vi "test Configuration File Read and Write.vi"(8 "error in (no error)":errorcluster, 11 "TestCase in":refnum<class "Configuration Tests.lvclass">) -> (0 "error out":errorcluster, 3 "TestCase out":refnum<class "Configuration Tests.lvclass">)   [LabVIEW 2017, in "Configuration Tests.lvclass"]
uses:
  Configuration Tests.lvclass
  Typedefs/DSF Engine Framework Configuration.ctl
  Typedefs/DSF Engine Plugin Configuration.ctl
  Typedefs/DSF Timing Info.ctl
  Typedefs/DSF Engine Plugin Thread Configuration.ctl
  Typedefs/DSF Settings Info.ctl
  Typedefs/DSF Engine Transfer Group Configuration.ctl
  Typedefs/DSF Direction.ctl
  Typedefs/DSF Engine Transfer Configuration.ctl
  Typedefs/DSF Byte Order.ctl
  Typedefs/DSF Engine Channel Configuration.ctl
  Typedefs/DSF Data Type.ctl
  Typedefs/DSF Timeout Behavior.ctl
  <vilib>/addons/_JKI Toolkits/VI Tester/TestCase.llb/TestCase.lvclass
  Classes/Configuration/Configuration Session.lvclass
  DSF Core.lvlib
  C:/Program Files (x86)/National Instruments/LabVIEW 2017/vi.lib/addons/_JKI Toolkits/VI Tester/TestCase.llb/TestCase.lvclass
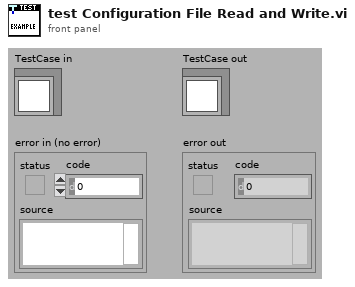
[diagram p1: front panel]
types:
  T1 = typedef "DSF Core.lvlib/DSF Engine Framework Configuration.ctl" = cluster{"Plugins":T2[]}
  T2 = typedef "DSF Core.lvlib/DSF Engine Plugin Configuration.ctl" = cluster{"name":string, "components":string[], "cycle timing":T3, "threads":T4[], "Transfer Groups":T6[], "settings":T5}
  T3 = typedef "DSF Core.lvlib/DSF Timing Info.ctl" = cluster{"priority":u64, "decimation":u64, "offset":u64}
  T4 = typedef "DSF Core.lvlib/DSF Engine Plugin Thread Configuration.ctl" = cluster{"buffer converter settings":T5, "transceiver settings":T5, "processor":i32, "priority offset":i16}
  T5 = typedef "DSF Core.lvlib/DSF Settings Info.ctl" = cluster{"key":string, "value":string}[]
  T6 = typedef "DSF Core.lvlib/DSF Engine Transfer Group Configuration.ctl" = cluster{"name":string, "direction":T7, "cycle timing":T3, "thread index":i32, "settings":T5, "Transfers":T8[], "timeout behavior":T12}
  T7 = typedef "DSF Core.lvlib/DSF Direction.ctl" = enum8{"Tx", "Rx"}
  T8 = typedef "DSF Core.lvlib/DSF Engine Transfer Configuration.ctl" = cluster{"name":string, "byte order":T9, "settings":T5, "channels":T10[]}
  T9 = typedef "DSF Core.lvlib/DSF Byte Order.ctl" = enum8{"big-endian", "little-endian"}
  T10 = typedef "DSF Core.lvlib/DSF Engine Channel Configuration.ctl" = cluster{"string offset":u64, "string data type":T11, "engine data type":T11, "name":string, "settings":T5, "units":string}
  T11 = typedef "DSF Core.lvlib/DSF Data Type.ctl" = enum8{"Bool", "SGL", "DBL", "I8", "I16", "I32", "I64", "U8", "U16", "U32", "U64"}
  T12 = typedef "DSF Core.lvlib/DSF Timeout Behavior.ctl" = enum8{"Increment Late Count", "Throw Error"}
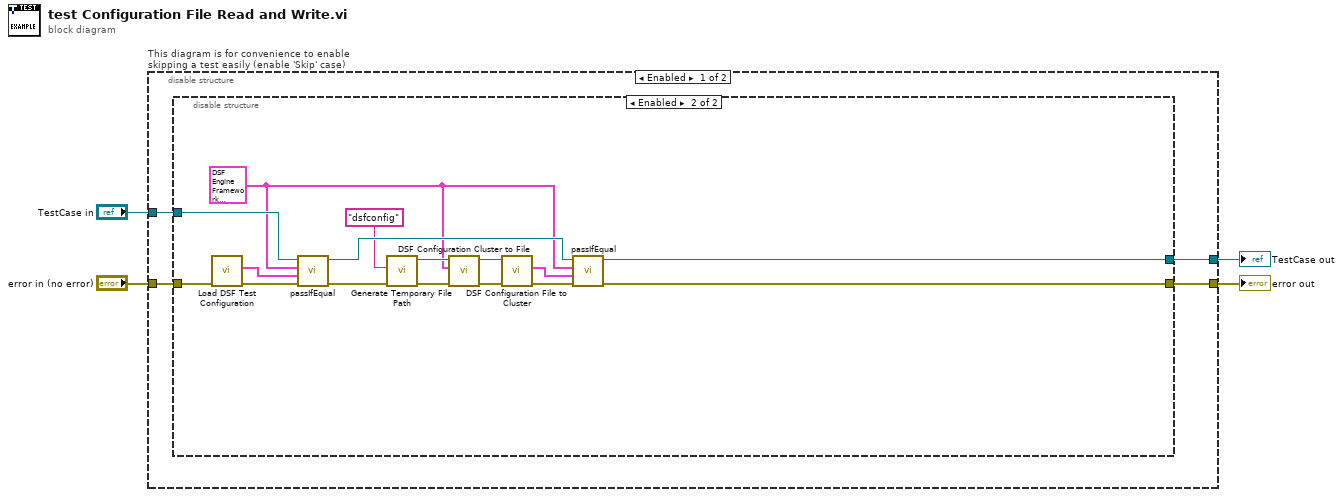
[diagram p0: block diagram]
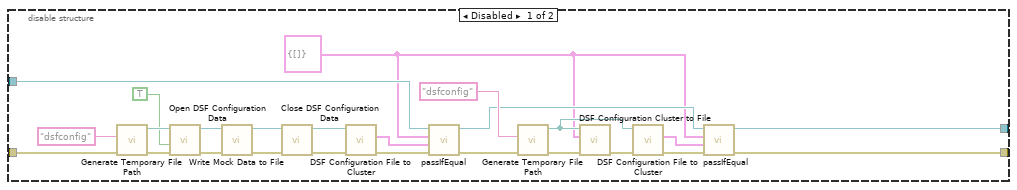
[diagram p2: hidden frame]
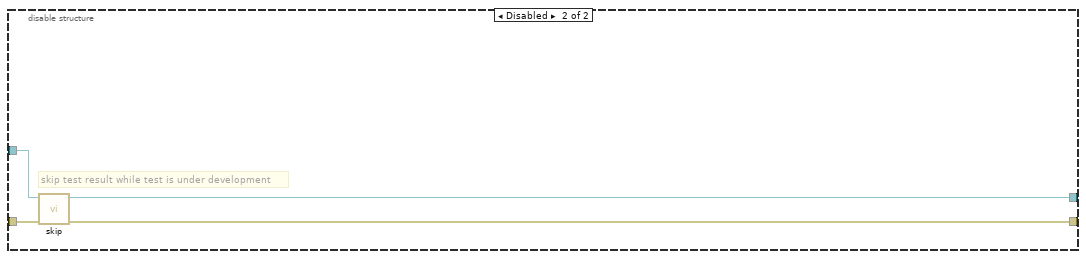
[diagram p3: hidden frame]
diagram:
  n1 = disable-structure "This diagram is for convenience to enable skipping a test easily (enable 'Skip' case)" shown="Enabled" {
    disable-tunnel: "TestCase in" -> [w7 w53]
    disable-tunnel: [w5 w51] -> w1
    disable-tunnel: [w6 w52] -> w3
    disable-tunnel: "error in (no error)" -> [w8 w50]
    frame Enabled {
      n2 = disable-structure shown="Enabled" {
        disable-tunnel: w8 -> [w33 w36]
        disable-tunnel: w7 -> [w24 w49]
        disable-tunnel: [w18 w46] -> w6
        disable-tunnel: [w16 w44] -> w5
        frame Disabled {
          w10 = T1 {"Plugins"=[]} ("framework configuration")
          n3 = call <vilib>:"Generate Temporary File Path.vi"("error in (no error)"=w33, "Temporary File Extension (tmp)"="dsfconfig") -> ("error out"=w32:errorcluster, "Unique Temporary File Path"=w31:path)  [unwired: 8 in]
          n4 = call "Open DSF Configuration Data.vi"("error in (no error)"=w32, "replace if found? (F)"=TRUE, "dsf configuration file path"=w31) -> ("error out"=w29:errorcluster, "Configuration Session"=w28:refnum<class "Configuration Session.lvclass">)  [unwired: 4 in, 3 out]
          n5 = call "Write Mock Data to File.vi"("error in (no error)"=w29, "Configuration Session in"=w28) -> ("error out"=w11:errorcluster, "Configuration Session out"=w27:refnum<class "Configuration Session.lvclass">)  [unwired: 8 in]
          n6 = call "Close DSF Configuration Data.vi"("error in (no error)"=w11, "Configuration Session"=w27) -> ("error out"=w26:errorcluster, "file path"=w19:path)  [unwired: 8 in]
          n7 = call "DSF Configuration File to Cluster.vi"("error in (no error)"=w26, "dsf configuration file path"=w19) -> ("error out"=w25:errorcluster, "framework configuration out"=w23:T1)  [unwired: 7 in, 1 out]
          n8 = call-dynamic "passIfEqual.vi"("error in (no error)"=w25, "y"=w23, "x"=w10, "TestCase in"=w24) -> ("error out"=w21:errorcluster, "TestCase out"=w17:refnum<class "Configuration Tests.lvclass">)  [unwired: 6 in]
          n9 = call <vilib>:"Generate Temporary File Path.vi"("error in (no error)"=w21, "Temporary File Extension (tmp)"="dsfconfig") -> ("error out"=w20:errorcluster, "Unique Temporary File Path"=w13:path)  [unwired: 8 in]
          n10 = call "DSF Configuration Cluster to File.vi"("error in (no error)"=w20, "framework configuration"=w10, "dsf configuration file path"=w13) -> ("error out"=w15:errorcluster)  [unwired: 7 in, 1 out]
          n11 = call "DSF Configuration File to Cluster.vi"("error in (no error)"=w15, "dsf configuration file path"=w13) -> ("error out"=w14:errorcluster, "framework configuration out"=w12:T1)  [unwired: 7 in, 1 out]
          n12 = call-dynamic "passIfEqual.vi"("error in (no error)"=w14, "y"=w12, "x"=w10, "TestCase in"=w17) -> ("error out"=w18:errorcluster, "TestCase out"=w16:refnum<class "Configuration Tests.lvclass">)  [unwired: 6 in]
        }
        frame Enabled {
          w39 = T1 {"Plugins"=[{"name"="UDP", "components"=["UDP"], "cycle timing"={"priority"=100, "decimation"=1, "offset"=0}, "threads"=[{"buffer converter settings"=[], "transceiver settings"=[{"key"="Local Port", "value"="50000"}], "processor"=-2, "priority offset"=0}, {"buffer converter settings"=[], "transceiver settings"=[{"key"="Local Port", "value"="50001"}], "processor"=-2, "priority offset"=0}, {"buffer converter settings"=[], "transceiver settings"=[{"key"="Local Port", "value"="50002"}], "processor"=-2, "priority offset"=0}, {"buffer converter settings"=[], "transceiver settings"=[{"key"="Local Port", "value"="50003"}], "processor"=-2, "priority offset"=0}], "Transfer Groups"=[{"name"="Group0", "direction"=enum."Tx", "cycle timing"={"priority"=100, "decimation"=1, "offset"=0}, "thread index"=0, "settings"=[], "Transfers"=[{"name"="Transfer0", "byte order"=enum."big-endian", "settings"=[{"key"="Destination Port", "value"="60000"}, {"key"="Destination Address", "value"="localhost"}], "channels"=[{"string offset"=0, "string data type"=enum."SGL", "engine data type"=enum."DBL", "name"="Temp", "settings"=[], "units"="V"}, {"string offset"=4, "string data type"=enum."DBL", "engine data type"=enum."DBL", "name"="RPM", "settings"=[], "units"="V"}, {"string offset"=12, "string data type"=enum."Bool", "engine data type"=enum."DBL", "name"="LED", "settings"=[], "units"="V"}, {"string offset"=792, "string data type"=enum."U64", "engine data type"=enum."DBL", "name"="Count", "settings"=[], "units"="V"}]}], "timeout behavior"=enum."Increment Late Count"}], "settings"=[]}]} ("framework configuration")
          n13 = call "Load DSF Test Configuration.vi"("error in (no error)"=w36) -> ("error out"=w35:errorcluster, "framework configuration"=w34:T1)  [unwired: 8 in, 1 out]
          n14 = call-dynamic "passIfEqual.vi"("error in (no error)"=w35, "y"=w34, "x"=w39, "TestCase in"=w49) -> ("error out"=w48:errorcluster, "TestCase out"=w45:refnum<class "Configuration Tests.lvclass">)  [unwired: 6 in]
          n15 = call <vilib>:"Generate Temporary File Path.vi"("error in (no error)"=w48, "Temporary File Extension (tmp)"="dsfconfig") -> ("error out"=w47:errorcluster, "Unique Temporary File Path"=w41:path)  [unwired: 8 in]
          n16 = call "DSF Configuration Cluster to File.vi"("error in (no error)"=w47, "framework configuration"=w39, "dsf configuration file path"=w41) -> ("error out"=w43:errorcluster, "dsf configuration file path dup"=w37:path)  [unwired: 7 in]
          n17 = call "DSF Configuration File to Cluster.vi"("error in (no error)"=w43, "dsf configuration file path"=w37) -> ("error out"=w42:errorcluster, "framework configuration out"=w40:T1)  [unwired: 7 in, 1 out]
          n18 = call-dynamic "passIfEqual.vi"("error in (no error)"=w42, "y"=w40, "x"=w39, "TestCase in"=w45) -> ("error out"=w46:errorcluster, "TestCase out"=w44:refnum<class "Configuration Tests.lvclass">)  [unwired: 6 in]
        }
      }
    }
    frame Disabled {
      # "skip test result while test is under development"
      n19 = call <vilib>:"skip.vi"("error in (no error)"=w50, "TestCase in"=w53) -> ("error out"=w52:errorcluster, "TestCase out"=w51:refnum<class "Configuration Tests.lvclass">)  [unwired: 8 in]
    }
  }
  "error out" <- w3
  "TestCase out" <- w1
